vi "Read Spectrum Analyzer.lvclass.vi"(11 "MCCW ACLR in":refnum<class "MCCW ACLR.lvclass">) -> (2 "Spectrum Analyzer.lvclass":refnum<class "Spectrum Analyzer.lvclass">, 3 "MCCW ACLR out":refnum<class "MCCW ACLR.lvclass">)   [LabVIEW 2020, in "MCCW ACLR.lvclass"]
uses:
  MCCW ACLR.lvclass
  Instruments/Spectrum Analyzer/Spectrum Analyzer.lvclass
  MCCW ACLR.lvclass/MCCW ACLR.ctl
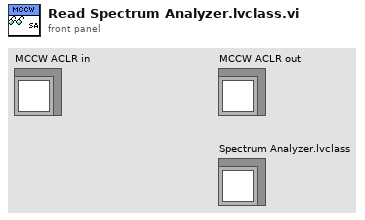
[diagram p1: front panel]
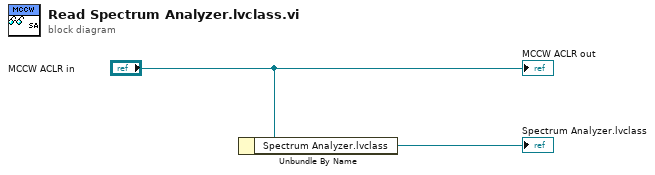
[diagram p0: block diagram]
diagram:
  n1 = Unbundle By Name("MCCW ACLR in") -> ("Spectrum Analyzer.lvclass"=→"Spectrum Analyzer.lvclass":refnum<class "Spectrum Analyzer.lvclass">)
  "MCCW ACLR out" <- "MCCW ACLR in"
